vi "position_variance.vi"(10 "feedback_time (ms)":fxp<+,16,1>, 11 "accn_noise":fxp<+,16,16>) -> (1 "E31":fxp<+,32,16>, 2 "E33":fxp<+,32,16>, 3 "E11":fxp<+,32,16>, 4 "output valid":bool)   [LabVIEW 2020]
uses:
  <vilib>/rvi/FXPMathLib/FxpMul/XNode/nifxpmath_Multiplier.xnode
  <vilib>/rvi/FXPMathLib/sim/FxpSim.dll
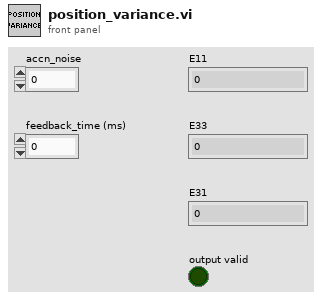
[diagram p1: front panel]
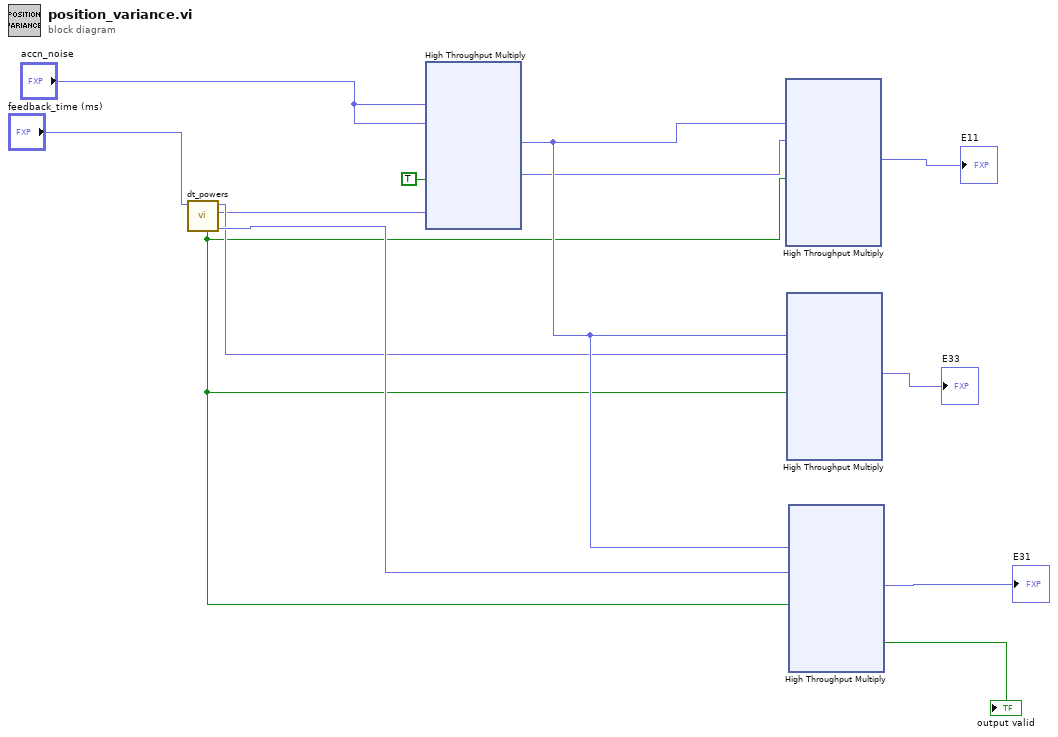
[diagram p0: block diagram]
diagram:
  n1 = call "dt_powers.vi"("feedback_time (ms)"="feedback_time (ms)") -> ("dt^3/2"=w9:fxp<+,48,1>, "dt^4/4"=w5:fxp<+,64,4>, "dt^2"=w7:fxp<+,32,2>, "output valid"=w2:bool)  [unwired: 6 in, 1 out]
  n2 = xnode ("High Throughput Multiply")("x"="accn_noise", "y"="accn_noise", "input valid"=TRUE) -> ("x*y"=w12:fxp<+,32,32>)  [unwired: 1 in, 2 out]
  n3 = xnode ("High Throughput Multiply")("x"=w12, "y"=w5, "input valid"=w2) -> ("x*y"=→"E11":fxp<+,32,16>)  [unwired: 1 in, 2 out]
  n4 = xnode ("High Throughput Multiply")("x"=w12, "y"=w7, "input valid"=w2) -> ("x*y"=→"E33":fxp<+,32,16>)  [unwired: 1 in, 2 out]
  n5 = xnode ("High Throughput Multiply")("x"=w12, "y"=w9, "input valid"=w2) -> ("x*y"=→"E31":fxp<+,32,16>, "output valid"=→"output valid":bool)  [unwired: 1 in, 1 out]
